vi "串口调试助手.vi"() -> ()   [LabVIEW 2020]
uses:
  <vilib>/Instr/_visa.llb/VISA Configure Serial Port (Instr).vi
panel:
  in  "ms/次":dbl
  in  "换行":bool
  in  "VISA resource name":refnum<visa-resource-name> caption="串口名"
  in  "stop bits (10: 1 bit)":u16(ring)=10 caption="停止位" items=["1.0"=10, "1.5"=15, "2.0"=20]
  in  "parity (0:none)":enum16{"None", "Odd", "Even", "Mark", "Space"}(ring) caption="校验位"
  in  "data bits (8)":u16(ring)=8 caption="数据位" items=["8"=8]
  in  "baud rate (9600)":u64(ring)=9600 caption="波特率" items=["9600"=9600, "18200"=18200, "38400"=38400, "115200"=115200]
  in  "时间循环开关":bool
  out "系统时间":string
  in  "清除接收":bool
  in  "时间戳":bool
  in  "HEX显示":bool
  in  "发送\n发送":bool
  in  "停止发送":bool
  in  "定时发送":bool
  in  "清除发送":bool
  in  "HEX发送":bool
  in  "发送区":string
  out "接收区":string
  in  "串口开关":bool
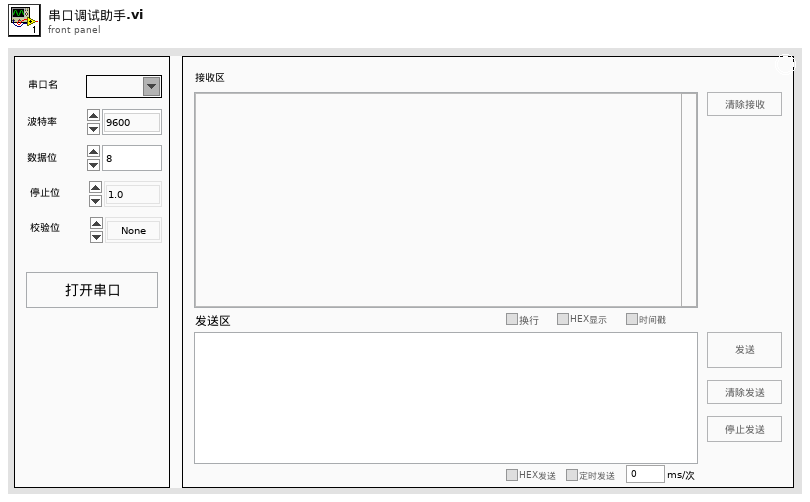
[diagram p1: front panel]
types:
  T1 = enum32{"invalid app kind", "Development System", "Run Time System", "Student Edition", "Embedded LabVIEW", "Evaluation", "Custom"}
  T2 = enum8{"Enabled", "Disabled", "Disabled and Grayed Out"}
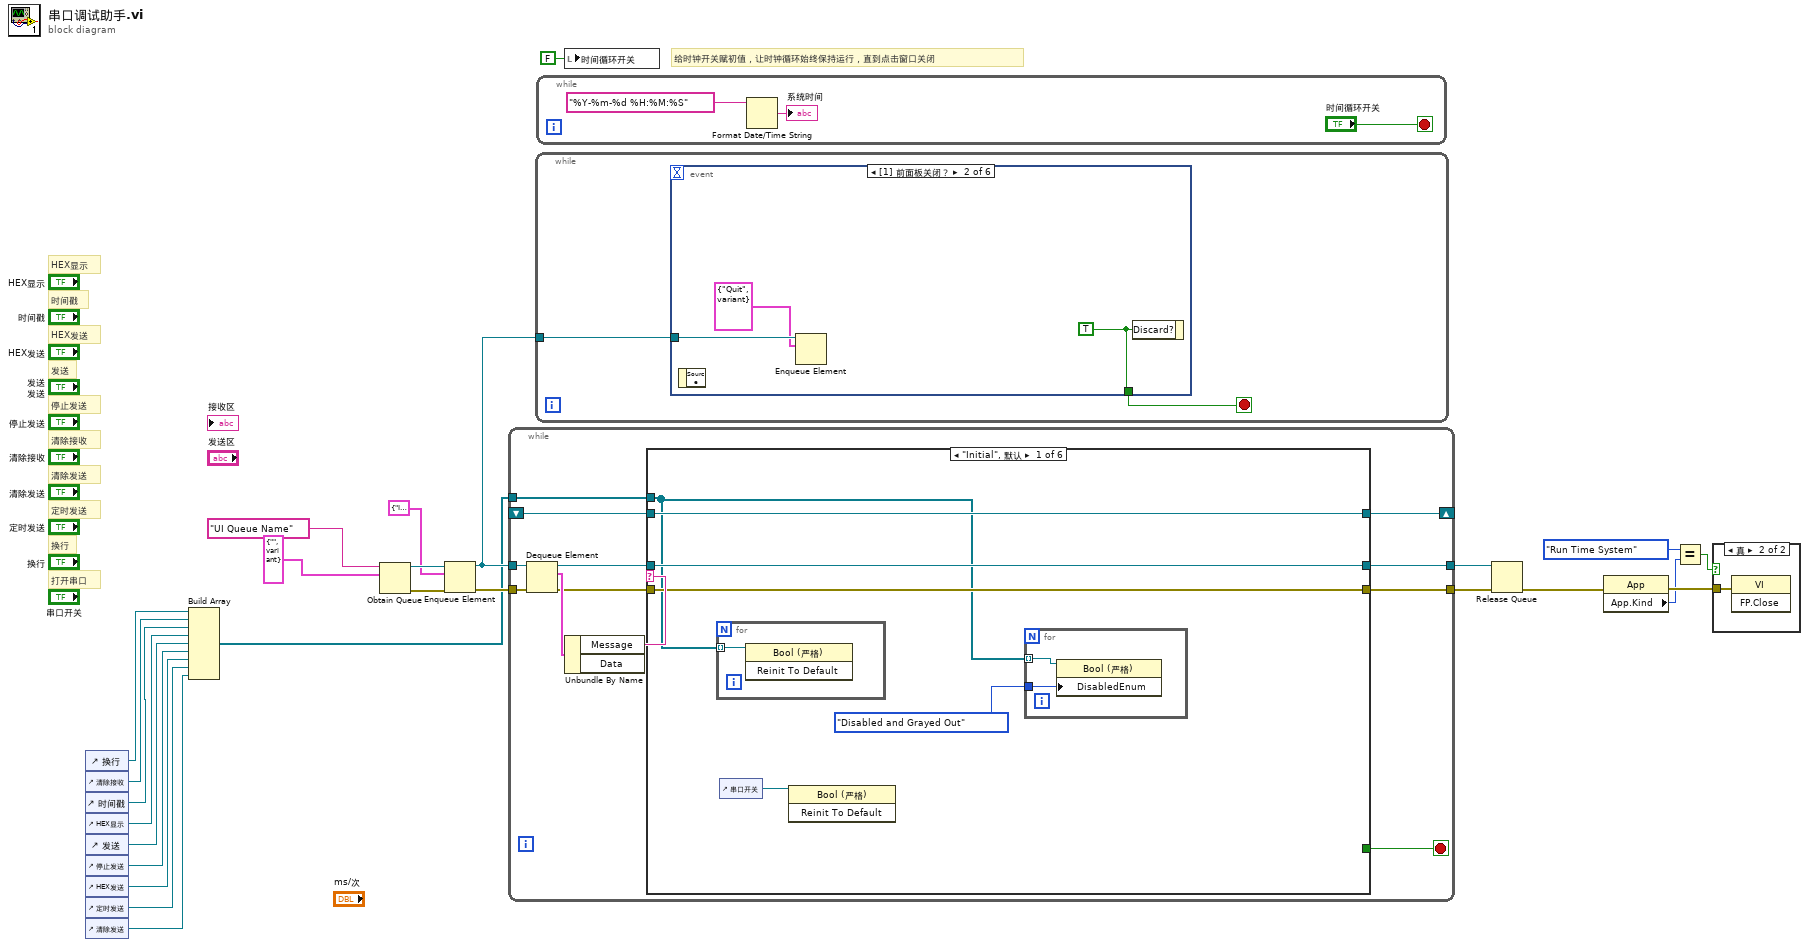
[diagram p0: block diagram]
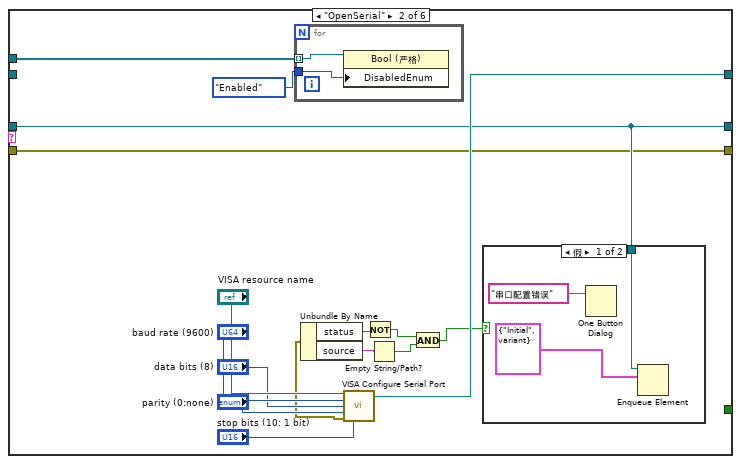
[diagram p3: hidden frame]
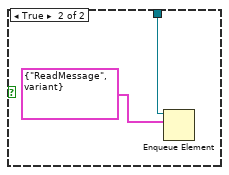
[diagram p4: hidden frame]
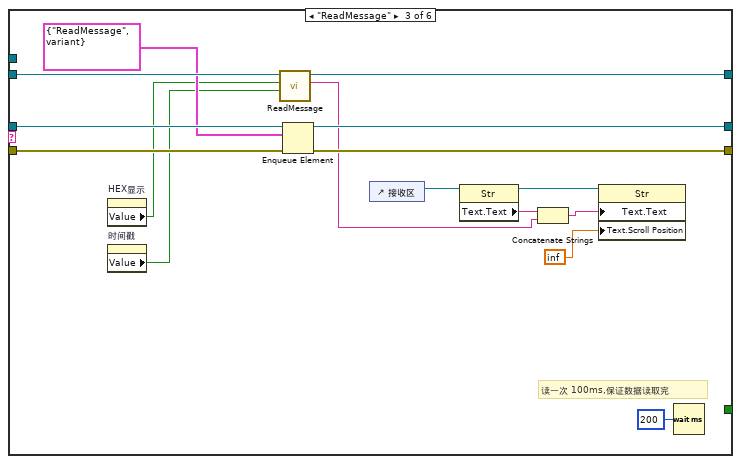
[diagram p5: hidden frame]
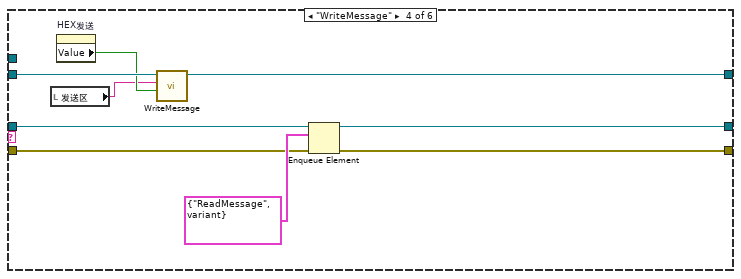
[diagram p6: hidden frame]
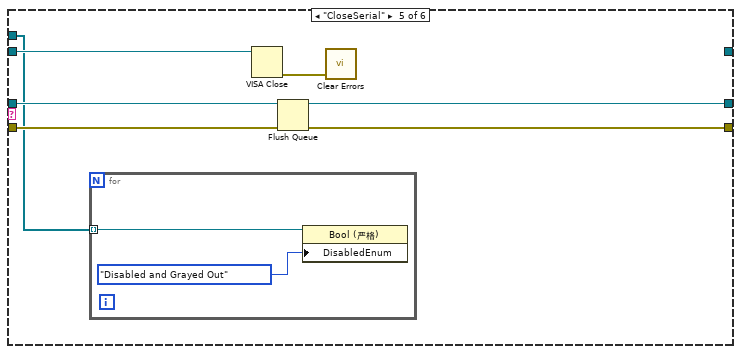
[diagram p7: hidden frame]
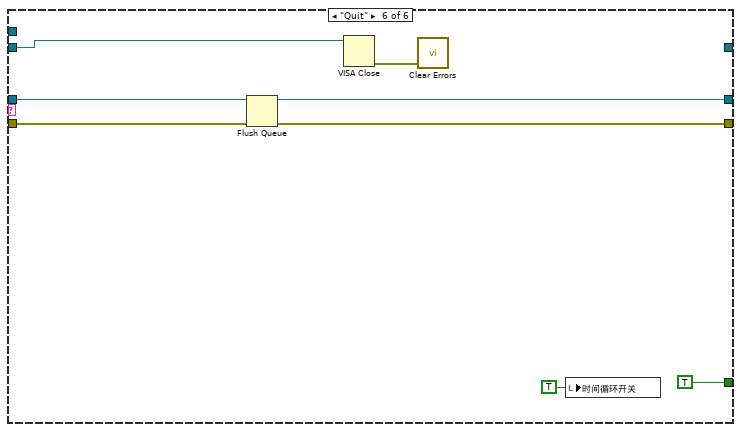
[diagram p8: hidden frame]
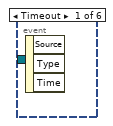
[diagram p9: hidden frame]
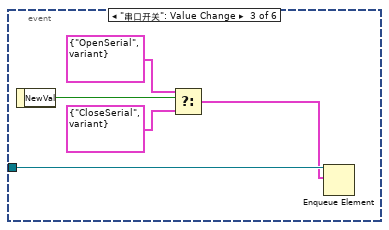
[diagram p10: hidden frame]
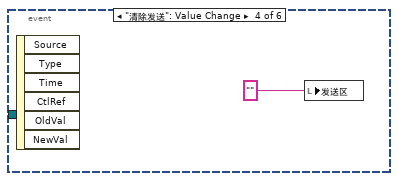
[diagram p11: hidden frame]
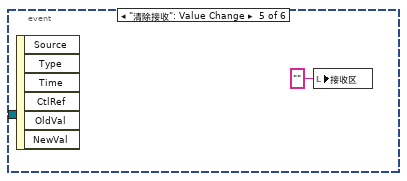
[diagram p12: hidden frame]
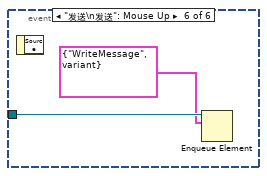
[diagram p13: hidden frame]
diagram:
  # "给时钟开关赋初值，让时钟循环始终保持运行，直到点击窗口关闭"
  # "换行"
  # "定时发送"
  # "打开串口"
  # "清除发送"
  # "清除接收"
  # "HEX显示"
  # "HEX发送"
  # "停止发送"
  # "发送"
  # "时间戳"
  n1 = control-ref of="换行"() -> (w3:refnum<vi>)
  n2 = control-ref of="清除接收"() -> (w4:refnum<vi>)
  n3 = control-ref of="时间戳"() -> (w5:refnum<vi>)
  n4 = control-ref of="HEX显示"() -> (w6:refnum<vi>)
  n5 = control-ref of="发送"() -> (w7:refnum<vi>)
  n6 = control-ref of="停止发送"() -> (w8:refnum<vi>)
  n7 = control-ref of="HEX发送"() -> (w9:refnum<vi>)
  n8 = control-ref of="定时发送"() -> (w10:refnum<vi>)
  n9 = control-ref of="清除发送"() -> (w11:refnum<vi>)
  n10 = Build Array(w3, w4, w5, w6, w7, w8, w9, w10, w11) -> (w2:refnum<vi>[])
  n11 = Obtain Queue(name (unnamed)="UI Queue Name" ("名称（未命名）"), element data type=cluster{"\nMessage":string, "\nData":variant} {"\nMessage"="", "\nData"=variant}) -> (queue out=w24:refnum<queue>, error out=w23:errorcluster)  [unwired: 3 in, 1 out]
  n12 = Enqueue Element(queue=w24, element=cluster{string, variant} {"Initial", variant}, error in (no error)=w23) -> (queue out=w12:refnum<queue>, error out=w20:errorcluster)  [unwired: 1 in, 1 out]
  n13 = while {
    tunnel: w12 -> [w37]
    tunnel: w20 -> [w36]
    shift-right: [w29] -> _
    shift-left: _ -> [w31]
    tunnel: [w28] -> w14
    tunnel: [w27] -> w13
    tunnel: w2 -> [w26]
    stop <- w30 stop-if-true
    n14 = Dequeue Element(queue=w37, error in (no error)=w36) -> (queue out=w33:refnum<queue>, element=w35:cluster{"\nMessage":string, "\nData":variant}, error out=w32:errorcluster)  [unwired: 1 in, 1 out]
    n15 = Unbundle By Name(w35) -> ("Message"=w34:string)  [unwired: 1 out]
    n16 = case shown="\"Initial\", 默认" w34 {
      tunnel: w33 -> [w43 w54 w83 w91 w99 w111]
      tunnel: w32 -> [w42 w53 w82 w88 w96 w110]
      tunnel: [w41 w62 w85 w93 _ _] -> w29
      tunnel: [w43 w54 w81 w90 w98 w108] -> w28
      tunnel: [w42 w53 w80 w89 w97 w107] -> w27
      tunnel: w31 -> [w41 _ w84 w94 w101 w105]
      tunnel: [_ _ _ _ _ TRUE] -> w30
      tunnel: w26 -> [w38 w47 _ _ w95 _]
      frame "Initial", Default {
        n17 = for {
          tunnel: w38 -> [w46] mode=indexing
          n18 = invoke class="Bool (严格)" method="Reinit To Default"(reference=w46) -> ()  [unwired: 2 in, 3 out]
        }
        n19 = control-ref of="串口开关"() -> (w39:refnum<vi>)
        n20 = invoke class="Bool (严格)" method="Reinit To Default"(reference=w39) -> ()  [unwired: 2 in, 3 out]
        n21 = for {
          tunnel: T2."Disabled and Grayed Out" ("禁用") -> [w45]
          tunnel: w38 -> [w44] mode=indexing
          n22 = property class="Bool (严格)"(reference=w44, "DisabledEnum"=w45) -> ()  [unwired: 1 in, 2 out]
        }
      }
      frame "OpenSerial" {
        n23 = for {
          tunnel: w47 -> [w64] mode=indexing
          tunnel: T2."Enabled" ("禁用") -> [w63]
          n24 = property class="Bool (严格)"(reference=w64, "DisabledEnum"=w63) -> ()  [unwired: 1 in, 2 out]
        }
        n25 = call-poly "VISA Configure Serial Port"("VISA resource name"="VISA resource name", "baud rate (9600)"="baud rate (9600)", "data bits (8)"="data bits (8)", "parity (0:none)"="parity (0:none)", "stop bits (10: 1 bit)"="stop bits (10: 1 bit)") -> ("VISA resource name out"=w62:refnum<visa-resource-name>, "error out"=w56:errorcluster)  [unwired: 9 in]
        n26 = Unbundle By Name(w56) -> ("status"=w55:bool, "source"=w52:string)
        n27 = Not(x=w55) -> (.not. x?=w51:bool)
        n28 = Empty String/Path?(string/path=w52) -> (empty?=w50:bool)
        n29 = And(x=w51, y=w50) -> (x .and. y?=w49:bool)
        n30 = case shown="假" w49 {
          tunnel: w54 -> [w66 w68]
          frame False {
            n31 = One Button Dialog(message="串口配置错误" ("消息")) -> ()  [unwired: 1 in, 1 out]
            n32 = Enqueue Element(queue=w66, element=cluster{string, variant} {"Initial", variant}) -> ()  [unwired: 2 in, 3 out]
          }
          frame True {
            n33 = Enqueue Element(queue=w68, element=cluster{string, variant} {"ReadMessage", variant}) -> ()  [unwired: 2 in, 3 out]
          }
        }
      }
      frame "ReadMessage" {
        # "读一次 100ms,保证数据读取完"
        n34 = property on="HEX显示" class="Bool (严格)"() -> ("Value"=w72:bool)  [unwired: 2 in, 2 out]
        n35 = property on="时间戳" class="Bool (严格)"() -> ("Value"=w71:bool)  [unwired: 2 in, 2 out]
        n36 = call "ReadMessage.vi"("时间戳"=w71, "HEX显示"=w72, "VISA资源名称"=w84) -> ("读取缓冲区"=w76:string, "VISA资源名称输出"=w85:refnum<visa-resource-name>)  [unwired: 7 in]
        n37 = Enqueue Element(queue=w83, element=cluster{"\nMessage":string, "\nData":variant} {"\nMessage"="ReadMessage", "\nData"=variant} ("元素"), error in (no error)=w82) -> (queue out=w81:refnum<queue>, error out=w80:errorcluster)  [unwired: 1 in, 1 out]
        n38 = control-ref of="接收区"() -> (w78:refnum<vi>)
        n39 = property class="Str"(reference=w78) -> (reference out=w75:refnum<vi>, "Text.Text"=w77:string)  [unwired: 1 in, 1 out]
        n40 = Concatenate Strings(w77, w76) -> (w74:string)
        n41 = property class="Str"(reference=w75, "Text.Text"=w74, "Text.Scroll Position"=inf) -> ()  [unwired: 1 in, 2 out]
        n42 = Wait (ms)(milliseconds to wait=u32 200 ("等待时间（毫秒）")) -> ()  [unwired: 1 out]
      }
      frame "WriteMessage" {
        n43 = local read "发送区"() -> (w86:string)
        n44 = property on="HEX发送" class="Bool (严格)"() -> ("Value"=w87:bool)  [unwired: 2 in, 2 out]
        n45 = call "WriteMessage.vi"("HEX发送"=w87, "写入缓冲区"=w86, "VISA资源名称"=w94) -> ("VISA资源名称输出"=w93:refnum<visa-resource-name>)  [unwired: 8 in]
        n46 = Enqueue Element(queue=w91, element=cluster{"\nMessage":string, "\nData":variant} {"\nMessage"="ReadMessage", "\nData"=variant} ("元素"), error in (no error)=w88) -> (queue out=w90:refnum<queue>, error out=w89:errorcluster)  [unwired: 1 in, 1 out]
      }
      frame "CloseSerial" {
        n47 = for {
          tunnel: w95 -> [w103] mode=indexing
          n48 = property class="Bool (严格)"(reference=w103, "DisabledEnum"=T2."Disabled and Grayed Out" ("禁用")) -> ()  [unwired: 1 in, 2 out]
        }
        n49 = VISA Close(VISA resource name=w101) -> (error out=w100:errorcluster)  [unwired: 1 in]
        n50 = Flush Queue(queue=w99, error in (no error)=w96) -> (queue out=w98:refnum<queue>, error out=w97:errorcluster)  [unwired: 1 out]
        n51 = call <vilib>:"Clear Errors.vi"("error in (no error)"=w100) -> ()  [unwired: 5 in, 2 out]
      }
      frame "Quit" {
        n52 = Flush Queue(queue=w111, error in (no error)=w110) -> (queue out=w108:refnum<queue>, error out=w107:errorcluster)  [unwired: 1 out]
        n53 = VISA Close(VISA resource name=w105) -> (error out=w106:errorcluster)  [unwired: 1 in]
        n54 = call <vilib>:"Clear Errors.vi"("error in (no error)"=w106) -> ()  [unwired: 5 in, 2 out]
        n55 = local write "时间循环开关"(TRUE ("时间循环开关")) -> ()
      }
    }
  }
  n56 = while {
    tunnel: w12 -> [w113]
    stop <- w112 stop-if-true
    n57 = event shown="[1] 前面板关闭？" {
      selector: _ -> [_ _ _ _ _ _]
      dyn-events: _ -> [_ _ _ _ _ _]
      timeout: _ -> [_ _ _ _ _ _]
      tunnel: [_ w116 _ _ _ _] -> w112
      tunnel: w113 -> [_ w115 w121 _ _ w125]
      event Timeout {
        n58 = event-data() -> ()  [unwired: 1 in, 3 out]
      }
      event Panel Close? {
        w116 = TRUE
        n59 = event-data() -> ()  [unwired: 1 in, 1 out]
        n60 = Enqueue Element(queue=w115, element=cluster{string, "元素":variant} {"Quit", "元素"=variant}) -> ()  [unwired: 2 in, 3 out]
        n61 = event-data("Discard?"=w116) -> ()  [unwired: 1 in, 1 out]
      }
      event "串口开关": Value Change {
        n62 = event-data() -> ("NewVal"=w120:bool)  [unwired: 1 in]
        n63 = Select(t=cluster{"\nMessage":string, "\nData":variant} {"\nMessage"="OpenSerial", "\nData"=variant} ("元素"), s=w120, f=cluster{"\nMessage":string, "\nData":variant} {"\nMessage"="CloseSerial", "\nData"=variant} ("元素")) -> (s? t:f=w117:cluster{"\nMessage":string, "\nData":variant})
        n64 = Enqueue Element(queue=w121, element=w117) -> ()  [unwired: 2 in, 3 out]
      }
      event "清除发送": Value Change {
        n65 = event-data() -> ()  [unwired: 1 in, 6 out]
        n66 = local write "发送区"("" ("接收区")) -> ()
      }
      event "清除接收": Value Change {
        n67 = event-data() -> ()  [unwired: 1 in, 6 out]
        n68 = local write "接收区"("" ("接收区")) -> ()
      }
      event "发送\n发送": Mouse Up {
        n69 = event-data() -> ()  [unwired: 1 in, 1 out]
        n70 = Enqueue Element(queue=w125, element=cluster{string, variant} {"WriteMessage", variant}) -> ()  [unwired: 2 in, 3 out]
      }
    }
  }
  n71 = while {
    stop <- "时间循环开关" stop-if-true
    n72 = Format Date/Time String(time format string (%c)="%Y-%m-%d %H:%M:%S" ("时间格式字符串(%c)")) -> (date/time string=→"系统时间":string)  [unwired: 2 in]
  }
  n73 = local write "时间循环开关"(FALSE ("时间循环开关")) -> ()
  n74 = Release Queue(queue=w14, error in (no error)=w13) -> (error out=w19:errorcluster)  [unwired: 1 in, 2 out]
  n75 = property class="App"(error in=w19) -> (error out=w17:errorcluster, "App.Kind"=w15:T1)  [unwired: 1 in, 1 out]
  n76 = Equal?(x=T1."Run Time System", y=w15) -> (x = y?=w18:bool)
  n77 = case shown="真" w18 {
    tunnel: w17 -> [_ w129]
    frame False {
    }
    frame True {
      n78 = invoke class="VI" method="FP.Close"(error in=w129) -> ()  [unwired: 2 in, 3 out]
    }
  }
